vi "Flight Gear Data RT Driver VI.vi"(10 "Device Outputs FIFO":refnum<k33>, 11 "Device Reference":T1 format="%.0x") -> ()   [LabVIEW 2010, in "Flight Gear Data Custom Device.lvlib"]
uses:
  Flight Gear Data Custom Device.lvlib
  <vilib>/NI VeriStand/Custom Device API/Custom Device Item Ref.ctl
  <vilib>/NI VeriStand/Custom Device API/Custom Device Channel Type.ctl
  FlightGearState.ctl
  <vilib>/NI VeriStand/Custom Device API/Get Item Property (U16).vi
  <vilib>/NI Veristand/Custom Device API/Custom Device API.lvlib
  <vilib>/NI Veristand/Custom Device Tools/Custom Device Utility Library/Custom Device Utility Library.lvlib
panel:
  in  "Status Notifier":refnum<notifier>
  # "Custom Device Template\nv1.0"
  # "Use this template as a starting point for creating a custom device code module. The input controls shown here are specially named controls that the system will use to provide the device loop with data. The controls are not required for the device loop to run. For instance, if the device doesn't produce any output data, then you don't need the Device Outputs FIFO control. If you do use these controls, however, they need to have these exact names to be functional."
  # "The optional status notifier element is used to notify the RT engine of the last state of the custom device, and to indicate the device has completed execution. If this control is not used, a default No Error value is returned to the system when the device finishes execution.\n\nNote: This error state is not checked until the system shuts down. Use an output status channel to send more immediate status values to the system."
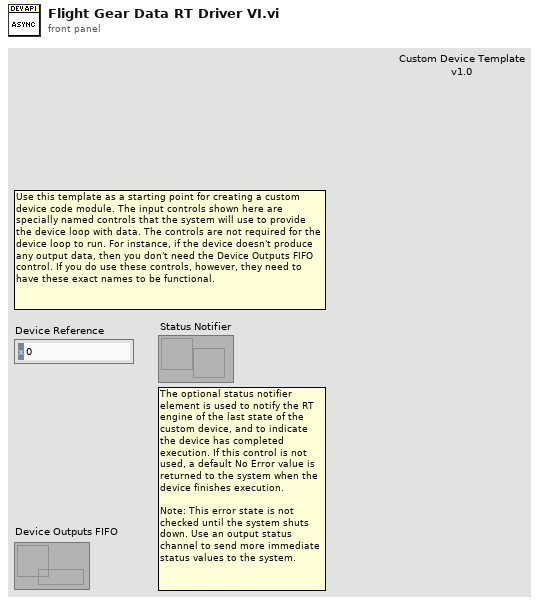
[diagram p1: front panel]
types:
  T1 = typedef "Custom Device API.lvlib/Custom Device Item Ref.ctl" = u64
  T2 = typedef "Flight Gear Data Custom Device.lvlib/FlightGearState.ctl" = enum16{"Initialize", "Read", "Write", "Close"}
  T3 = typedef "Custom Device API.lvlib/Custom Device Channel Type.ctl" = enum16{"Input", "Output"}
  T4 = typedef "Flight Gear Data Custom Device.lvlib/FGNetFDM.ctl" = cluster{"Version":cluster{"version":u32, "pad":u32}, "Positions":cluster{"Doubles":cluster{"longitude":dbl, "latitude":dbl, "altitude":dbl}, "Singles":cluster{"agl":sgl, "phi":sgl, "theta":sgl, "psi":sgl, "alpha":sgl, "beta":sgl}}, "Velocities":cluster{"phidot":sgl, "thetadot":sgl, "psidot":sgl, "vcas":sgl, "climb_rate":sgl, "v_north":sgl, "v_east":sgl, "v_down":sgl, "v_wind_body_north":sgl, "v_wind_body_east":sgl, "v_wind_body_down":sgl}, "Accelerations":cluster{"A_X_pilot":sgl, "A_Y_pilot":sgl, "A_Z_pilot":sgl}, "Stall":cluster{"stall_warning":sgl, "slip_deg":sgl}, "Engine Status":cluster{"num_engines":u32, "eng_state":u32[], "rpm":sgl[], "fuel_flow":sgl[], "fuel_px":sgl[], "egt":sgl[], "cht":sgl[], "mp_osi":sgl[], "tit":sgl[], "oil_temp":sgl[], "oil_px":sgl[]}, "Consumables":cluster{"num_tanks":u32, "fuel_quantity":sgl[]}, "Gear Status":cluster{"num_wheels":u32, "wow":u32[], "gear_pos":sgl[], "gear_steer":sgl[], "gear_compression":sgl[]}, "Environment":cluster{"curr_time":u32, "warp":i32, "visibility":sgl}, "Control Surface Positions":cluster{"elevator":sgl, "elevator_trim_tab":sgl, "left_flap":sgl, "right_flap":sgl, "left aileron":sgl, "right_aileron":sgl, "rudder":sgl, "nose_wheel":sgl, "speedbrake":sgl, "spoilers":sgl}}
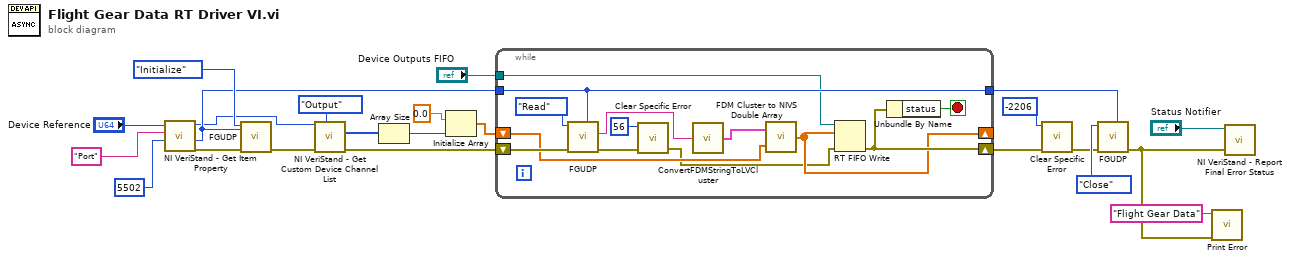
[diagram p0: block diagram]
diagram:
  n1 = call-poly <vilib>:"NI VeriStand - Get Item Property.vi"("Default Value"=u16 5502 ("Remote Port"), "Property Name"="Port", "Item Ref in"="Device Reference") -> ("error out"=w7:errorcluster, "Value"=w8:u16, "Item Ref out"=w1:T1)  [unwired: 5 in, 1 out]
  n2 = call "FGUDP.vi"("Port"=w8, "Error In"=w7, "UDP State"=FlightGearState."Initialize") -> ("error out"=w15:errorcluster)  [unwired: 7 in, 1 out]
  n3 = call <vilib>:"NI VeriStand - Get Custom Device Channel List.vi"("Channel Type"=Custom_Device_Channel_Type."Output", "error in (no error)"=w15, "Device Ref in"=w1) -> ("error out"=w23:errorcluster, "Specified Channel Ref List"=w18:T1[])  [unwired: 7 out]
  n4 = Array Size(array=w18) -> (size(s)=w17:i32)
  n5 = Initialize Array(0.0 ("element"), w17) -> (w20:dbl[])
  n6 = while {
    shift-right: [w27] -> _
    shift-left: w20 -> [w25]
    shift-right: [w32] -> w6
    shift-left: w23 -> [w34]
    tunnel: "Device Outputs FIFO" -> [w33]
    tunnel: w8 -> [w36]
    tunnel: [w36] -> w12
    stop <- w31 stop-if-true
    n7 = call "FGUDP.vi"("Port"=w36, "Error In"=w34, "UDP State"=FlightGearState."Read") -> ("error out"=w30:errorcluster, "Data String Out"=w28:string)  [unwired: 7 in]
    n8 = call "Clear Specific Error.vi"("error in (no error)"=w30, "code"=56) -> ("error out"=w24:errorcluster)  [unwired: 9 in]
    n9 = call "ConvertFDMStringToLVCluster.vi"("FGNetFDM"=w28) -> ("Cluster"=w26:T4)
    n10 = call "FDM Cluster to NIVS Double Array.vi"("Buffer In"=w25, "Cluster"=w26) -> ("DBL Array"=w27:dbl[])
    n11 = RT FIFO Write(0:w33, 1:w27, 3:w24) -> (11:w32:errorcluster)  [unwired: 2 in, 3 out]
    n12 = Unbundle By Name(w32) -> ("status"=w31:bool)
  }
  n13 = call "Clear Specific Error.vi"("error in (no error)"=w6, "code"=-2206) -> ("error out"=w5:errorcluster)  [unwired: 9 in]
  n14 = call "FGUDP.vi"("Port"=w12, "Error In"=w5, "UDP State"=FlightGearState."Close") -> ("error out"=w3:errorcluster)  [unwired: 7 in, 1 out]
  n15 = call "Print Error.vi"("error out"=w3, "Your code's public name"="Flight Gear Data") -> ()  [unwired: 9 in]
  n16 = call <vilib>:"NI VeriStand - Report Final Error Status.vi"("error in (no error)"=w3, "Status Notifier"="Status Notifier") -> ()  [unwired: 1 in, 9 out]
